vi "RSZVB Get Converter Source Frequency.vi"(8 "error in (no error)":errorcluster {"code" format="%.0x"}, 9 "Port (1)":i32=1, 10 "Channel (1)":i32=1, 11 "VISA session":refnum<visa-resource-name>) -> (0 "error out":errorcluster {"code" format="%.0x"}, 1 "Numerator":i32, 3 "dup VISA session":refnum<visa-resource-name>, 4 "Sweep Type":i32, 5 "Offset":dbl format="%^.3e", 7 "Denominator":i32)   [LabVIEW 2011]
doc: "This VI returns the converter source frequency at the converter port <Pt>.\n\nNotes:\n\n(1) This command is available for frequency converters with electronic attenuators R&S ZVA-ZxxxE.\n\nRemote-control command(s):\nSOURce<Ch>:FREQuency<Pt>:CONVersion:ARBitrary:CFRequency?"
uses:
  _utility/RSZVB Global Data.vi
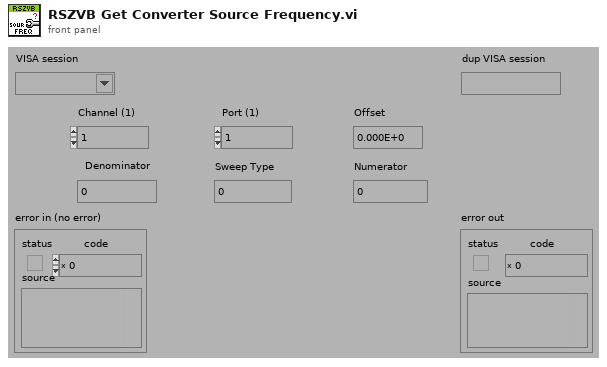
[diagram p1: front panel]
types:
  T1 = cluster{"Error Checking (T: On)":bool, "Installed Options":string[], "Data Valid?":bool, "Ports":i32, "Model":string[], "Option Checking (T: On)":bool}[]
  T2 = cluster{"Error Checking (T: On)":bool, "Installed Options":string[], "Data Valid?":bool, "Ports":i32, "Model":string[], "Option Checking (T: On)":bool}
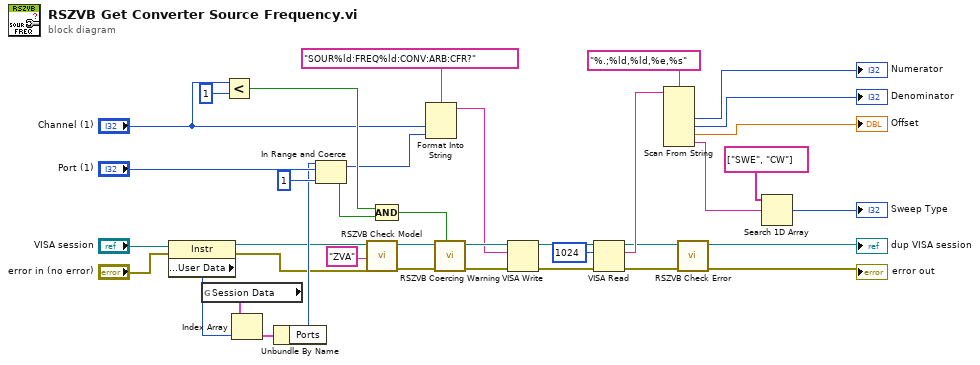
[diagram p0: block diagram]
diagram:
  n1 = property class="Instr"(reference="VISA session", error in="error in (no error)") -> (reference out=w25:refnum<visa-resource-name>, error out=w26:errorcluster, "General Settings:User Data"=w35:u32)
  n2 = global read "RSZVB Global Data.vi" "Session Data"() -> (w36:T1)
  n3 = Less?(x="Channel (1)", y=1) -> (x < y?=w27:bool)
  n4 = Index Array(array=w36, index=w35) -> (element=w37:T2)
  n5 = Unbundle By Name(w37) -> ("Ports"=w30:i32)
  n6 = In Range and Coerce(upper limit=w30, x="Port (1)", lower limit=1) -> (coerced(x)=w19:i32, In Range?=w28:bool)
  n7 = call "RSZVB Check Model.vi"("error in (no error)"=w26, "Model"="ZVA", "VISA session"=w25) -> ("error out"=w24:errorcluster, "dup VISA session"=w23:refnum<visa-resource-name>)  [unwired: 7 in]
  n8 = Compound Arithmetic op=AND(w27, w28) -> (w22:bool)
  n9 = Format Into String(format string="SOUR%ld:FREQ%ld:CONV:ARB:CFR?", "Channel (1)", w19) -> (resulting string=w16:string)  [unwired: 2 in, 1 out]
  n10 = call "RSZVB Coercing Warning.vi"("In Range?"=w22, "error in (no error)"=w24, "VISA session"=w23) -> ("error out"=w18:errorcluster, "dup VISA session"=w17:refnum<visa-resource-name>)  [unwired: 7 in]
  n11 = VISA Write(VISA resource name=w17, write buffer=w16, error in (no error)=w18) -> (VISA resource name out=w14:refnum<visa-resource-name>, error out=w15:errorcluster)  [unwired: 1 out]
  n12 = VISA Read(VISA resource name=w14, byte count=u32 1024, error in (no error)=w15) -> (VISA resource name out=w4:refnum<visa-resource-name>, read buffer=w11:string, error out=w3:errorcluster)  [unwired: 1 out]
  n13 = Scan From String(format string="%.;%ld,%ld,%e,%s", input string=w11) -> (output 1=→"Numerator":i32, output 2=→"Denominator":i32, output 3=→"Offset":dbl, output 4=w7:string)  [unwired: 6 in, 3 out]
  n14 = call "RSZVB Check Error.vi"("error in (no error)"=w3, "VISA session"=w4) -> ("error out"=→"error out":errorcluster, "dup VISA session"=→"dup VISA session":refnum<visa-resource-name>)  [unwired: 8 in]
  n15 = Search 1D Array(1D array=string[] ["SWE", "CW"], element=w7) -> (index of element=→"Sweep Type":i32)  [unwired: 1 in]
